vi "Initialize MeasurementLink Session.vi"(7 "remote connection options":T2, 8 "error in":errorcluster, 9 "initialize session behavior":T1, 10 "session initialization parameters":T3, 11 "instrument in":refnum<class "Instrument.lvclass">) -> (0 "error out":errorcluster, 2 "session out":variant, 3 "instrument out":refnum<class "Instrument.lvclass">)   [LabVIEW 2020, in "Keysight 34401A DMM Instrument.lvlib" / "Instrument.lvclass"]
uses:
  Instrument.lvclass
  Instrument.lvclass/Instrument.ctl
  <vilib>/MeasurementLink/MeasurementLink Measurement Server/Helpers/Error Strings Global Internal.vi
  <instrlib>/Agilent 34401/Agilent 34401.lvlib
  <vilib>/MeasurementLink/MeasurementLink Instrument/IInstrument/Initialize and Close Session Behavior.ctl
  <vilib>/MeasurementLink/MeasurementLink Instrument/IInstrument/IInstrument.lvclass
  <vilib>/MeasurementLink/MeasurementLink Instrument/IInstrument/Remote Connection Options.ctl
  <vilib>/MeasurementLink/MeasurementLink Instrument/IInstrument/Session Initialization Parameters.ctl
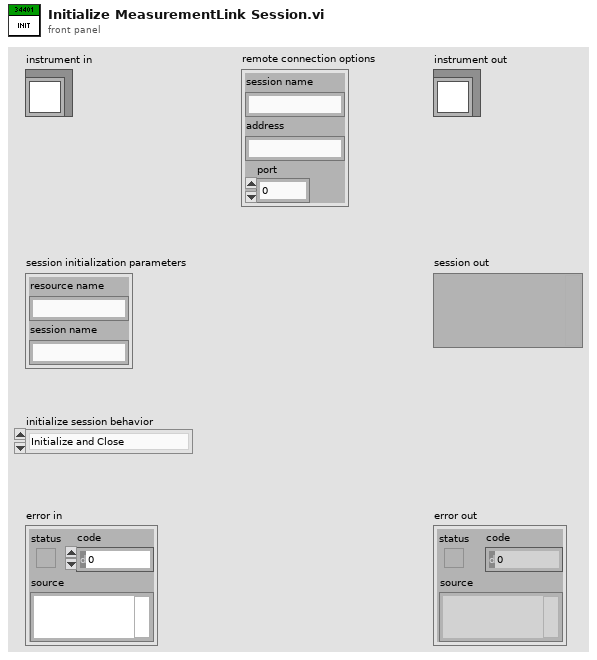
[diagram p1: front panel]
types:
  T1 = typedef "MeasurementLink Instrument.lvlib/IInstrument.lvclass/Initialize and Close Session Behavior.ctl" = enum16{"Initialize and Close", "Attach and Detach", "Initialize and Detach", "Attach and Close"}
  T2 = typedef "MeasurementLink Instrument.lvlib/IInstrument.lvclass/Remote Connection Options.ctl" = cluster{"session name":string, "address":string, "port":u32}
  T3 = typedef "MeasurementLink Instrument.lvlib/IInstrument.lvclass/Session Initialization Parameters.ctl" = cluster{"resource name":string, "session name":string}
  T4 = cluster{"Baud Rate":u32, "Parity":u16, "Data Bits":u16}
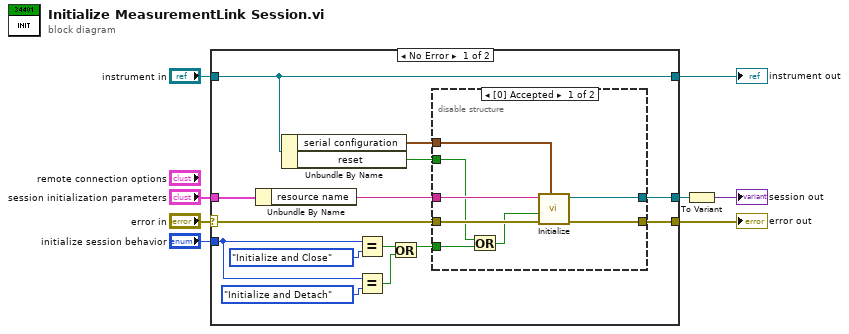
[diagram p0: block diagram]
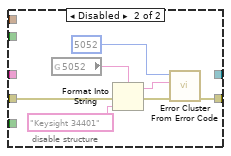
[diagram p2: hidden frame]
diagram:
  n1 = case shown="No Error" "error in" {
    selector: "error in" -> [w21 w38]
    tunnel: [w20 w38] -> w7
    tunnel: "instrument in" -> [w18 w39]
    tunnel: [w18 w39] -> w5
    tunnel: "initialize session behavior" -> [w10 _]
    tunnel: "session initialization parameters" -> [w19 _]
    tunnel: [w22 _] -> w2
    frame No Error {
      n2 = Unbundle By Name(w19) -> ("resource name"=w9:string)
      n3 = Unbundle By Name(w18) -> ("serial configuration"=w17:T4, "reset"=w15:bool)
      n4 = Equal?(x=w10, y=Initialize_and_Close_Session_Behavior."Initialize and Close" ("initialize session behavior")) -> (x = y?=w12:bool)
      n5 = Equal?(x=w10, y=Initialize_and_Close_Session_Behavior."Initialize and Detach" ("initialize session behavior")) -> (x = y?=w11:bool)
      n6 = Or(x=w12, y=w11) -> (x .or. y?=w14:bool)
      n7 = disable-structure shown="[0] Accepted" {
        disable-tunnel: [w30 _] -> w22
        disable-tunnel: w21 -> [w29 w31]
        disable-tunnel: [w28 w32] -> w20
        disable-tunnel: w9 -> [w27 _]
        disable-tunnel: w17 -> [w24 _]
        disable-tunnel: w14 -> [w26 _]
        disable-tunnel: w15 -> [w23 _]
        frame Enabled {
          n8 = Or(x=w23, y=w26) -> (x .or. y?=w25:bool)
          n9 = call <instrlib>:"Initialize.vi"("Serial Configuration"=w24, "error in (no error)"=w29, "Reset (True)"=w25, "VISA resource name"=w27) -> ("error out"=w28:errorcluster, "VISA resource name out"=w30:refnum<visa-resource-name>)  [unwired: 6 in]
        }
        frame Disabled {
          n10 = global read "Error Strings Global Internal.vi" "5052"() -> (w36:string)
          n11 = Format Into String(format string=w36, error in=w31, "Keysight 34401") -> (resulting string=w33:string, error out=w34:errorcluster)  [unwired: 1 in]
          n12 = call <vilib>:"Error Cluster From Error Code.vi"("error in (no error)"=w34, "error message (\"\")"=w33, "error code (0)"=5052) -> ("error out"=w32:errorcluster)  [unwired: 6 in]
        }
      }
    }
    frame Error {
    }
  }
  "error out" <- w7
  "instrument out" <- w5
  n13 = To Variant(anything=w2) -> (Variant=→"session out":variant)
